vi "Get Legend Axis.vi"(8 "error in (no error)":errorcluster, 11 "3D Ribbon in":refnum<class "3D Ribbon.lvclass">) -> (0 "error out":errorcluster, 1 "Active Axis":enum16{"X-axis", "Y-axis", "Z-axis"}(ring)=enum."Z-axis", 3 "3D Ribbon out":refnum<class "3D Ribbon.lvclass">)   [LabVIEW 2020, in "3D Ribbon.lvclass"]
uses:
  <vilib>/Math Plots/3D Math Plots/3D Ribbon/3D Ribbon/3D Ribbon.lvclass
  e:/builds/penguin/labview/branches/2020/dev/dist/vi.lib/Math Plots/3D Math Plots/3D Plot/3D Plot/3D Plot.lvclass
  <vilib>/Math Plots/3D Math Plots/3D Ribbon/3D Ribbon/3D Ribbon.lvclass/3D Ribbon.ctl
  <vilib>/Math Plots/3D Math Plots/3D Plot/3D Plot/3D Plot.lvclass
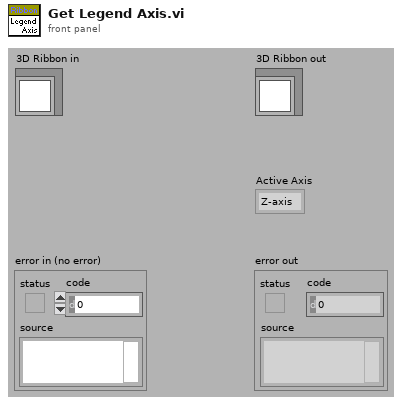
[diagram p1: front panel]
types:
  T1 = typedef "3D Ribbon.lvclass/3D Ribbon Property Array.ctl" = T2[]
  T2 = typedef "3D Ribbon.lvclass/3D Ribbon Property.ctl" = cluster{"General Property":cluster{"Plot Name":string, "Coordinate System":enum16{"Cartesian", "Cylindrical", "Spherical"}, "Opacity":sgl}, "Projection Property":cluster{"Draw XY":bool, "Draw YZ":bool, "Draw XZ":bool}, "Plot Property":cluster{"Draw Surface":bool, "Color Ramp Cluster":T3, "Line Style":T4, "Line Width":sgl, "Line Color":u32, "Antialiasing":bool}, "Ribbon Property":cluster{"Ribbon Mode":enum16{"Row", "Column"}, "Ribbon Width":sgl}}
  T3 = typedef "3D Plot.lvclass/Color Ramp Cluster.ctl" = cluster{"Color Ramp Style":enum16{"None", "Shaded", "Color spectrum", "Grey scale", "Custom"}, "Color Ramp Array":u32[], "Color Ramp Index":i32[], "Interpolate?":bool, "Logarithm?":bool}
  T4 = typedef "3D Plot.lvclass/Line Type.ctl" = enum16{"None", "Solid", "Dash", "Dot", "Dash Dot"}
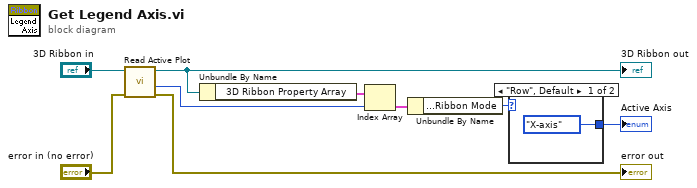
[diagram p0: block diagram]
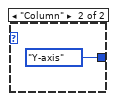
[diagram p2: hidden frame]
diagram:
  n1 = call <vilib>:"Read Active Plot.vi"("error in (no error)"="error in (no error)", "3D Plot.lvclass in"="3D Ribbon in") -> ("error out"=→"error out":errorcluster, "Active Plot"=w6:i32, "3D Plot.lvclass out"=w8:refnum<class "3D Ribbon.lvclass">)  [unwired: 7 out]
  "3D Ribbon out" <- w8
  n2 = Unbundle By Name(w8) -> ("3D Ribbon Property Array"=w7:T1)
  n3 = Index Array(array=w7, index=w6) -> (element=w5:T2)
  n4 = Unbundle By Name(w5) -> ("Ribbon Property.Ribbon Mode"=w4:enum16{"Row", "Column"})
  n5 = case shown="\"Row\", Default" w4 {
    tunnel: [enum16{"X-axis", "Y-axis", "Z-axis"}."X-axis" ("Active Axis") enum16{"X-axis", "Y-axis", "Z-axis"}."Y-axis" ("Active Axis")] -> w3
    frame "Row", Default {
    }
    frame "Column" {
    }
  }
  "Active Axis" <- w3
